vi "Autonomous.vi"(8 "Error In":errorcluster) -> (0 "Error Out":errorcluster, 2 "Switch To Teleop":bool)   [LabVIEW 2013]
panel:
  in  "Autonomous Comment":bool
  out "Top Goal":dbl
  out "Bottom  Goal":dbl
  in  "Was the goal lit?":string(combo)="No"
  in  "Did they move?":string(combo)="No" caption="Did they move out of the white zone?"
  in  "SWITCH TO TELEOP":bool
  in  "Autonomous?":string(combo)="No"
  in  "Did they start in \nthe goalie zone?":string(combo)="No"
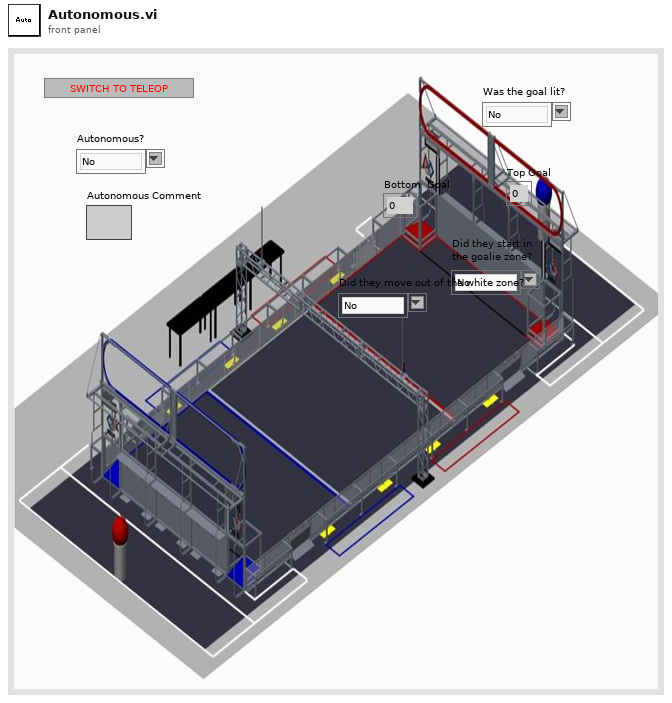
[diagram p1: front panel]
types:
  T1 = cluster{"Autonomous?":string, "Did they start in \nthe goalie zone?":string, "Did they move?":string, "Was the goal lit?":string}
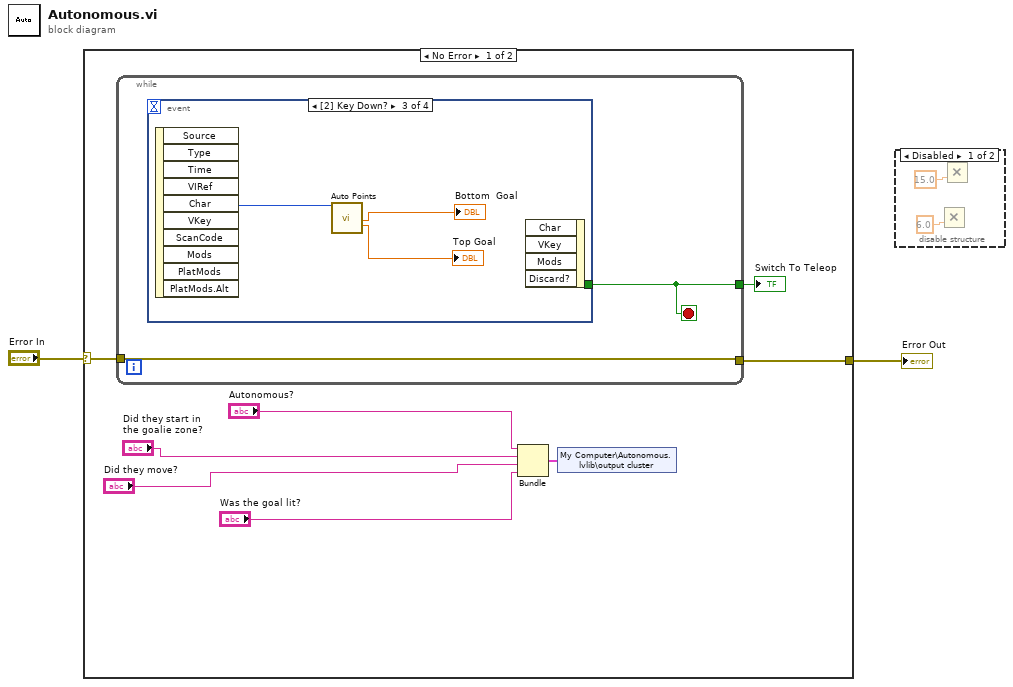
[diagram p0: block diagram]
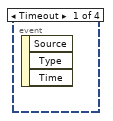
[diagram p3: hidden frame]
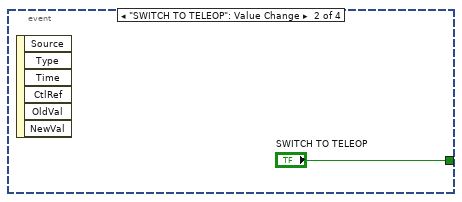
[diagram p4: hidden frame]
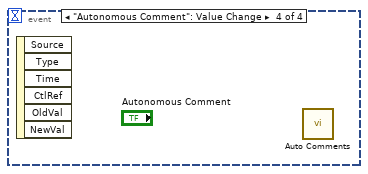
[diagram p5: hidden frame]
diagram:
  n1 = case shown="No Error" "Error In" {
    selector: "Error In" -> [w9 w17]
    tunnel: [w8 w17] -> w1
    frame No Error {
      n2 = while {
        tunnel: [w11] -> w10
        tunnel: [w12] -> w8
        tunnel: w9 -> [w12]
        stop <- w11 stop-if-true
        n3 = event shown="[2] Key Down?" {
          selector: _ -> [_ _ _ _]
          dyn-events: _ -> [_ _ _ _]
          timeout: _ -> [_ _ _ _]
          tunnel: [_ "SWITCH TO TELEOP" _ _] -> w11
          event Timeout {
            n4 = event-data() -> ()  [unwired: 1 in, 3 out]
          }
          event "SWITCH TO TELEOP": Value Change {
            n5 = event-data() -> ()  [unwired: 1 in, 6 out]
          }
          event Key Down? {
            n6 = event-data() -> ("Char"=w16:i16)  [unwired: 1 in, 9 out]
            n7 = call "Auto Points.vi"("Char"=w16) -> ("Bottom Goal"=→"Bottom  Goal":dbl, "Top Goal"=→"Top Goal":dbl)  [unwired: 16 in, 1 out]
            n8 = event-data() -> ()  [unwired: 5 in, 1 out]
          }
          event "Autonomous Comment": Value Change {
            n9 = event-data() -> ()  [unwired: 1 in, 6 out]
            n10 = call "Auto Comments.vi"() -> ()  [unwired: 11 in, 1 out]
          }
        }
      }
      "Switch To Teleop" <- w10
      n11 = Bundle("Autonomous?"="Autonomous?", "Did they start in \nthe goalie zone?"="Did they start in \nthe goalie zone?", "Did they move?"="Did they move?", "Was the goal lit?"="Was the goal lit?") -> (w3:T1)  [unwired: 1 in]
      n12 = shared-variable "My Computer\\Autonomous.lvlib\\output cluster"(w3) -> ()  [unwired: 1 in, 1 out]
    }
    frame Error {
    }
  }
  "Error Out" <- w1
  n13 = disable-structure shown="Disabled" {
    frame Disabled {
      n14 = Multiply(y=6.0) -> ()  [unwired: 1 in, 1 out]
      n15 = Multiply(y=15.0) -> ()  [unwired: 1 in, 1 out]
    }
    frame Enabled {
    }
  }
